vi "Segment Average.vi"(2 "Num Points":i32, 7 "New Point":dbl) -> (4 "Mean":dbl, 8 "Stdev":dbl, 15 "New Mean":bool)   [LabVIEW 2020]
uses:
  <vilib>/Analysis/NI_AALBase.lvlib
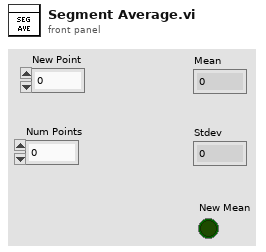
[diagram p1: front panel]
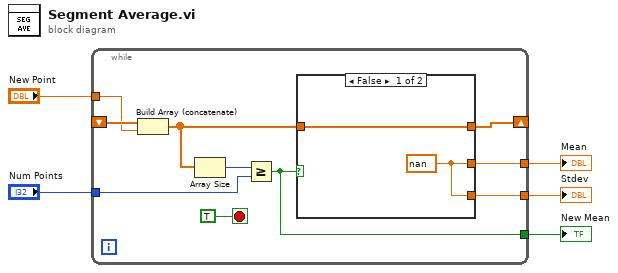
[diagram p0: block diagram]
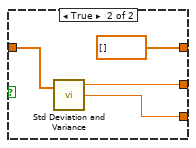
[diagram p2: hidden frame]
diagram:
  n1 = while {
    shift-right: [w14] -> _
    shift-left: _ -> [w12]
    tunnel: "New Point" -> [w11]
    tunnel: "Num Points" -> [w13]
    tunnel: [w8] -> w3
    tunnel: [w7] -> w2
    tunnel: [w6] -> w1
    stop <- TRUE stop-if-true
    n2 = Build Array (concatenate)(w12, w11) -> (w9:dbl[])
    n3 = Array Size(array=w9) -> (size(s)=w10:i32)
    n4 = Greater Or Equal?(x=w10, y=w13) -> (x >= y?=w6:bool)
    n5 = case shown="False" w6 {
      tunnel: [w17 dbl[] []] -> w14
      tunnel: w9 -> [w17 w20]
      tunnel: [w16 w19] -> w8
      tunnel: [w16 w18] -> w7
      frame False {
        w16 = nan ("mean")
      }
      frame True {
        n6 = call <vilib>:"Std Deviation and Variance.vi"("X"=w20) -> ("mean"=w19:dbl, "standard deviation"=w18:dbl)  [unwired: 1 in, 1 out]
      }
    }
  }
  "Mean" <- w3
  "New Mean" <- w1
  "Stdev" <- w2
